vi "dfd_Lattice Allpass Normalization (Norm).vi"(7 "scale type":T1, 10 "coefficients k":dbl[](array[numeric]) format="%.2f", 11 "x":dbl[](array[numeric])) -> (2 "norm":dbl[](array[numeric]) format="%.2f", 3 "y":dbl[](array[numeric]))   [LabVIEW 2017, in "NI_DigFilter_FXP.lvlib"]
uses:
  <vilib>/addons/Digital Filter Design/NI_DigFilter_FXP.lvlib
  <vilib>/addons/Digital Filter Design/_Objects.llb/DFD Coef Norm Type.ctl
  <vilib>/addons/Digital Filter Design/NI_DigFilterLicensed.lvlib
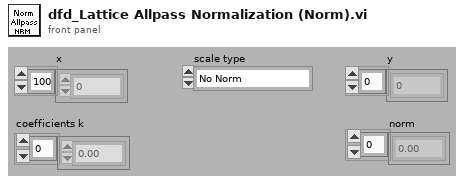
[diagram p1: front panel]
types:
  T1 = typedef "NI_DigFilterLicensed.lvlib/DFD Coef Norm Type.ctl" = enum16{"No Norm", "Time Domain 1-Norm", "Time Domain 2-Norm", "Time Domain Inf-Norm"}
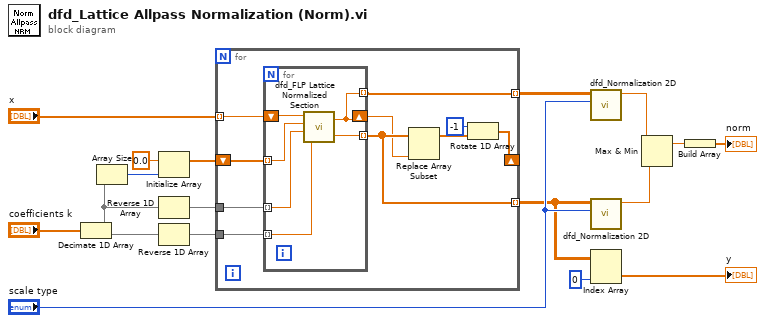
[diagram p0: block diagram]
diagram:
  n1 = Decimate 1D Array("coefficients k") -> (w6:dbl[], w5:dbl[])
  n2 = Array Size(array=w6) -> (size(s)=w17:i32)
  n3 = Initialize Array(0.0 ("element"), w17) -> (w18:dbl[])
  n4 = Reverse 1D Array(array=w6) -> (reversed array=w16:dbl[])
  n5 = Reverse 1D Array(array=w5) -> (reversed array=w4:dbl[])
  n6 = for {
    tunnel: w16 -> [w28]
    shift-right: [w27] -> _
    shift-left: w18 -> [w26]
    tunnel: [w24] -> w8 mode=indexing
    tunnel: [w25] -> w13 mode=indexing
    tunnel: "x" -> [w20] mode=indexing
    tunnel: w4 -> [w19]
    n7 = for {
      shift-right: [w31] -> w23
      shift-left: w20 -> [w30]
      tunnel: w26 -> [w34] mode=indexing
      tunnel: w28 -> [w33] mode=indexing
      tunnel: [w32] -> w24 mode=indexing
      tunnel: [w31] -> w25 mode=indexing
      tunnel: w19 -> [w29] mode=indexing
      n8 = call <vilib>:"dfd_FLP Lattice Normalized Section.vi"("^k(m)"=w29, "k(m)"=w33, "w(m-1)"=w34, "x(m)"=w30) -> ("w(m)"=w32:dbl, "x(m-1)"=w31:dbl)
    }
    n9 = Replace Array Subset(array=w24, new element=w23) -> (w22:dbl[])  [unwired: 1 in]
    n10 = Rotate 1D Array(1:w22, 2:-1 ("n")) -> (0:w27:dbl[])
  }
  n11 = call <vilib>:"dfd_Normalization 2D.vi"("scale type"="scale type", "2D Array (col-major)"=w13) -> ("max norm"=w11:dbl)  [unwired: 9 out]
  n12 = call <vilib>:"dfd_Normalization 2D.vi"("scale type"="scale type", "2D Array (col-major)"=w8) -> ("max norm"=w12:dbl)  [unwired: 9 out]
  n13 = Index Array(array=w8, index (col)=0 ("disabled index (col)")) -> (element=→"y":dbl[])  [unwired: 1 in]
  n14 = Max & Min(x=w11, y=w12) -> (max(x,y)=w10:dbl)  [unwired: 1 out]
  n15 = Build Array(w10) -> (→"norm":dbl[])
